vi "Test First Enqueued Return Value is Returned.vi"(8 "error in (no error)":errorcluster, 11 "Test Case In":refnum<class "Return Value Test.lvclass">) -> (0 "error out":errorcluster, 3 "Test Case Out":refnum<class "Return Value Test.lvclass">)   [LabVIEW 2020, in "Return Value Test.lvclass"]
uses:
  Return Value Test.lvclass
  C:/Program Files (x86)/National Instruments/LabVIEW 2020/vi.lib/Astemes/LUnit/Test Case.lvclass
  <vilib>/Astemes/LUnit/Test Case.lvclass/Test Case.ctl
  4993e8ee-a06a-463a-9684-69129f64d5ce.vi
  <vilib>/Astemes/LUnit/Append Pass Result.vi
  <vilib>/Astemes/LUnit/Append Fail Result.vi
  <vilib>/Astemes/LUnit/Describe Comparison.vi
  <vilib>/Astemes/LUnit/Compare Variants.vi
  <vilib>/Astemes/LUnit/Variant to string.vi
  <vilib>/Utility/Data Type/Get Type Information.vi
  <vilib>/Utility/LVClass/Get LV Class Name.vi
  Test Doubles/Test Interface Responsive Mock/Test Interface Mock.lvclass
  Return Value Test.lvclass/Return Value Test.ctl
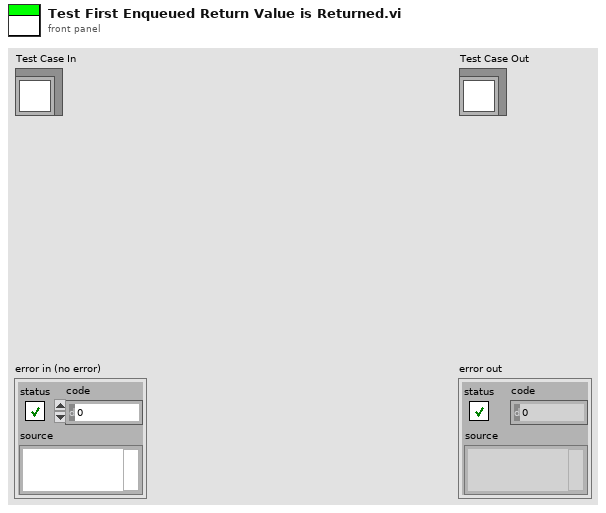
[diagram p1: front panel]
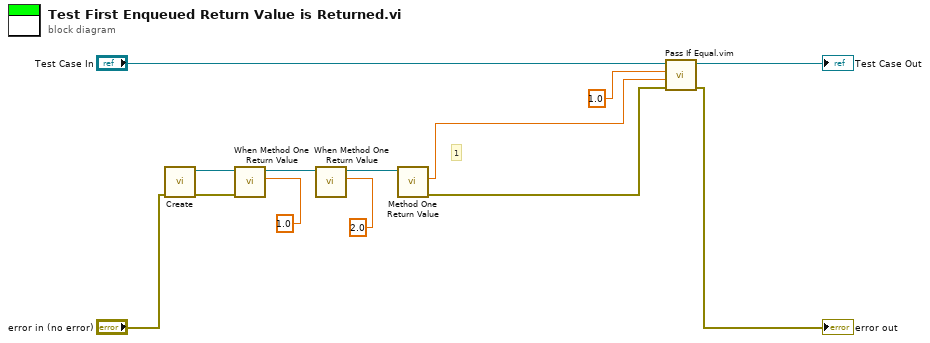
[diagram p0: block diagram]
diagram:
  # "1"
  n1 = call "Create.vi"("error in (no error)"="error in (no error)") -> ("error out"=w9:errorcluster, "Test Interface Mock Out"=w10:refnum<class "Test Interface Mock.lvclass">)  [unwired: 9 in]
  n2 = call "When Method One Return Value.vi"("Return Value"=1.0, "error in (no error)"=w9, "Test Interface Mock In"=w10) -> ("Test Interface Mock Out"=w8:refnum<class "Test Interface Mock.lvclass">)  [unwired: 8 in]
  n3 = call "When Method One Return Value.vi"("Return Value"=2.0, "Test Interface Mock In"=w8) -> ("Test Interface Mock Out"=w5:refnum<class "Test Interface Mock.lvclass">)  [unwired: 9 in]
  n4 = call-dynamic "Method One Return Value.vi"("Test Interface Mock in"=w5) -> ("error out"=w7:errorcluster, "Return Value"=w1:dbl)  [unwired: 8 in, 1 out]
  n5 = call "Pass If Equal.vim"("error in (no error)"=w7, "Actual"=w1, "Expected"=1.0 ("Return Value"), "LUnit Test Case In"="Test Case In") -> ("error out"=→"error out":errorcluster, "LUnit Test Case Out"=→"Test Case Out":refnum<class "Return Value Test.lvclass">)  [unwired: 6 in]
